vi "Report.vi"(9 "Report Elements":refnum<class>[](array[class]), 10 "Action Data":T1, 11 "Report Handler":refnum<class "Report Handler.lvclass">) -> (0 "error out":errorcluster)   [LabVIEW 2020, in "ProjectBuilder.lvlib" / "Report Handler.lvclass"]
uses:
  Report Handler.lvclass
  Ctl/Ctl_Action Data.ctl
  Report Data/Report Data.lvclass
  ProjectBuilder.lvlib
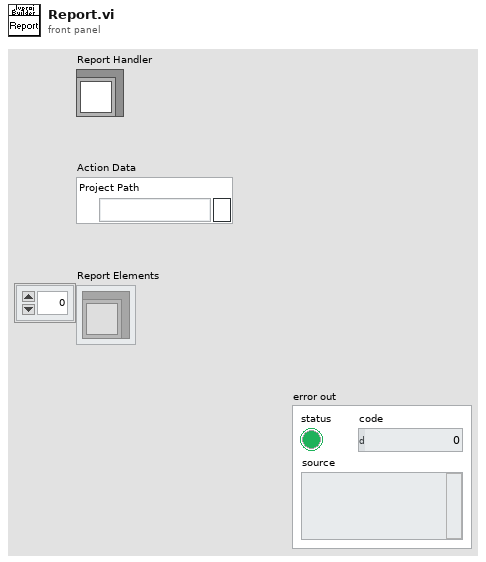
[diagram p1: front panel]
types:
  T1 = typedef "ProjectBuilder.lvlib/Ctl_Action Data.ctl" = cluster{"Project Path":path}
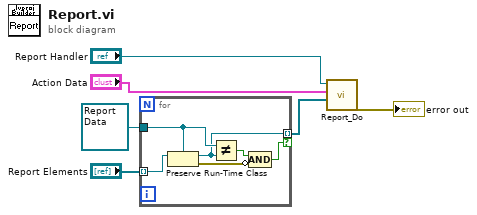
[diagram p0: block diagram]
diagram:
  n1 = for {
    tunnel: "Report Elements" -> [w12] mode=indexing
    tunnel: refnum<class "Report Data.lvclass"> refnum ("ProjectBuilder.lvlib:Report Interface.lvclass") -> [w11]
    tunnel: [w8] -> w4 mode=indexing if=w7
    n2 = Preserve Run-Time Class(object in=w12, 2:w11) -> (object out=w8:refnum<class "Report Data.lvclass">, error out=w9:errorcluster)  [unwired: 1 in]
    n3 = Not Equal?(x=w11, y=w8) -> (x != y?=w10:bool)
    n4 = Compound Arithmetic op=AND(w10, invert w9) -> (w7:bool)
  }
  n5 = call "Report_Do.vi"("Array"=w4, "Action Data"="Action Data", "Report Handler in"="Report Handler") -> ("error out"=→"error out":errorcluster)  [unwired: 8 in]
